vi "Lift Cycles.vi"(8 "liftMot":bool, 10 "changeDesired":bool) -> ()   [LabVIEW 2014]
uses:
  Robot Global Data.vi
  <vilib>/Rock Robotics/Network Tables/SD Write Number.vi
panel:
  in  "Desired Encoder In":dbl
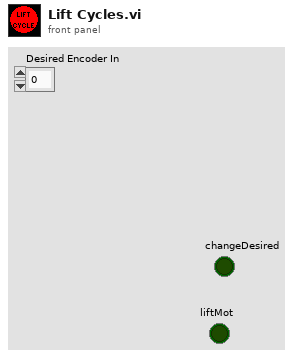
[diagram p1: front panel]
types:
  T1 = typedef "WPI_EncoderDevRef.ctl" = cluster{"DevStatus":errorcluster, "EncoderIndex":T2, "CounterIndex":T3, "DistancePerCount":dbl, "Decoding Type":T4}
  T2 = typedef "FPGA_EncoderIdx.ctl" = enum8{"Enc 0", "Enc 1", "Enc 2", "Enc 3", "Enc 4", "Enc 5", "Enc 6", "Enc 7", "Invalid"}
  T3 = typedef "FPGA_CounterCtrSystemIndex.ctl" = enum8{"Ctr 0", "Ctr 1", "Ctr 2", "Ctr 3", "Ctr 4", "Ctr 5", "Ctr 6", "Ctr 7", "Invalid"}
  T4 = typedef "WPI_EncoderType.ctl" = enum16{"1x", "2x", "4x"}
  T5 = typedef "WPI_MotorControlDeviceRef.ctl" = cluster{"DeviceStatus":errorcluster, "Type":T6, "PWM":cluster{"Controller":T7, "PWM Channel":T8, "DeadBand":T9}, "CAN":cluster{"Device Number":u8, "Control Mode":T10, "Semaphore":T11, "Max Vout":dbl, "TalonSRX Control Mode":T12}, "Invert":bool, "TransformRef":T13, "InvTransformRef":T13}
  T6 = typedef "WPI_MotorControlType.ctl" = enum16{"PWM", "CAN", "CANTalonSRX"}
  T7 = typedef "FPGA_TypedefDigitalModule.ctl" = enum16{"Controller 1"}
  T8 = typedef "FPGA_DIOPWMChannel.ctl" = enum8{"PWM 0", "PWM 1", "PWM 2", "PWM 3", "PWM 4", "PWM 5", "PWM 6", "PWM 7", "PWM 8", "PWM 9", "PWM MXP 0", "PWM MXP 1", "PWM MXP 2", "PWM MXP 3", "PWM MXP 4", "PWM MXP 5", "PWM MXP 6", "PWM MXP 7", "PWM MXP 8", "PWM MXP 9", "Invalid"}
  T9 = typedef "WPI_PWMDeadband.ctl" = cluster{"Name":string, "maxPositivePwm":i32, "minPositivePwm":i32, "centerPwm":i32, "maxNegativePwm":i32, "minNegativePwm":i32, "angularRange":u16}
  T10 = typedef "WPI_CANJaguar_ControlMode.ctl" = enum8{"Percent VBus", "Current", "Speed", "Position", "Voltage"}
  T11 = typedef "Semaphore RefNum" = refnum<k1>
  T12 = typedef "WPI_CANTalonSRX_APIControlMode.ctl" = enum8{"Percent VBus", "Speed", "Position", "Slave", "Unchanged / Invalid"}
  T13 = typedef "WPI_PWMTransform_ConPane.ctl" = refnum<vi>
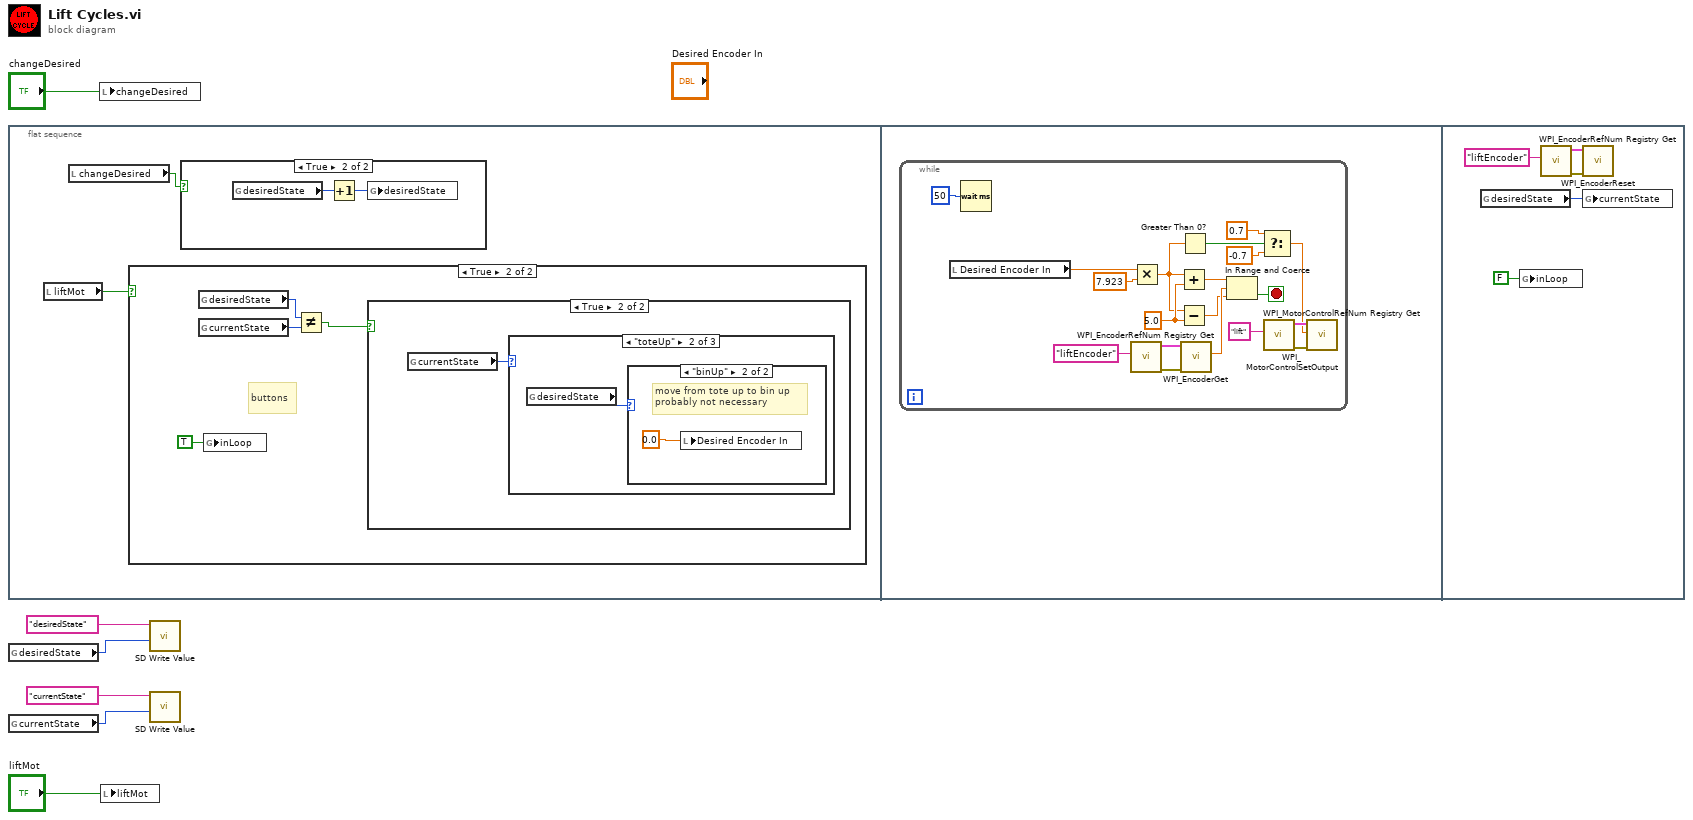
[diagram p0: block diagram]
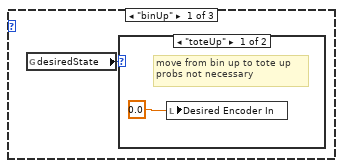
[diagram p4: hidden frame]
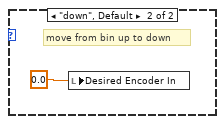
[diagram p5: hidden frame]
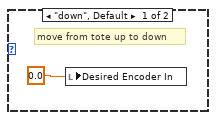
[diagram p6: hidden frame]
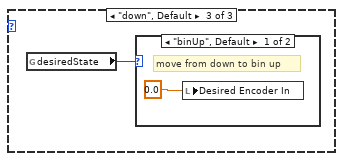
[diagram p7: hidden frame]
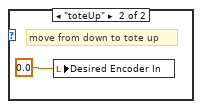
[diagram p8: hidden frame]
diagram:
  n1 = flat-sequence {
    frame #0 {
      n2 = local read "liftMot"() -> (w7:bool)
      n3 = local read "changeDesired"() -> (w8:bool)
      n4 = case shown="True" w7 {
        frame False {
        }
        frame True {
          # "buttons"
          n5 = global read "Robot Global Data.vi" "desiredState"() -> (w11:enum16{"binUp", "toteUp", "down"})
          n6 = global read "Robot Global Data.vi" "currentState"() -> (w12:enum16{"binUp", "toteUp", "down"})
          n7 = global write "Robot Global Data.vi" "inLoop"(TRUE) -> ()
          n8 = Not Equal?(x=w11, y=w12) -> (x != y?=w9:bool)
          n9 = case shown="True" w9 {
            frame False {
            }
            frame True {
              n10 = global read "Robot Global Data.vi" "currentState"() -> (w13:enum16{"binUp", "toteUp", "down"})
              n11 = case shown="\"toteUp\"" w13 {
                frame "binUp" {
                  n12 = global read "Robot Global Data.vi" "desiredState"() -> (w14:enum16{"binUp", "toteUp", "down"})
                  n13 = case shown="\"toteUp\"" w14 {
                    frame "toteUp" {
                      # "move from bin up to tote up\nprobs not necessary"
                      n14 = local write "Desired Encoder In"(0.0 ("Desired Encoder Clicks 2")) -> ()
                    }
                    frame "down", Default {
                      # "move from bin up to down"
                      n15 = local write "Desired Encoder In"(0.0 ("Desired Encoder Clicks 2")) -> ()
                    }
                  }
                }
                frame "toteUp" {
                  n16 = global read "Robot Global Data.vi" "desiredState"() -> (w17:enum16{"binUp", "toteUp", "down"})
                  n17 = case shown="\"binUp\"" w17 {
                    frame "down", Default {
                      # "move from tote up to down"
                      n18 = local write "Desired Encoder In"(0.0 ("Desired Encoder Clicks 2")) -> ()
                    }
                    frame "binUp" {
                      # "move from tote up to bin up\nprobably not necessary"
                      n19 = local write "Desired Encoder In"(0.0 ("Desired Encoder Clicks 2")) -> ()
                    }
                  }
                }
                frame "down", Default {
                  n20 = global read "Robot Global Data.vi" "desiredState"() -> (w20:enum16{"binUp", "toteUp", "down"})
                  n21 = case shown="\"binUp\", Default" w20 {
                    frame "binUp", Default {
                      # "move from down to bin up"
                      n22 = local write "Desired Encoder In"(0.0 ("Desired Encoder Clicks 2")) -> ()
                    }
                    frame "toteUp" {
                      # "move from down to tote up"
                      n23 = local write "Desired Encoder In"(0.0 ("Desired Encoder Clicks 2")) -> ()
                    }
                  }
                }
              }
            }
          }
        }
      }
      n24 = case shown="True" w8 {
        frame False {
        }
        frame True {
          n25 = global read "Robot Global Data.vi" "desiredState"() -> (w23:enum16{"binUp", "toteUp", "down"})
          n26 = Increment(x=w23) -> (x+1=w24:enum16{"binUp", "toteUp", "down"})
          n27 = global write "Robot Global Data.vi" "desiredState"(w24) -> ()
        }
      }
    }
    frame #1 {
      n28 = while {
        stop <- w36 stop-if-true
        w38 = 5.0 ("y")
        n29 = local read "Desired Encoder In"() -> (w25:dbl)
        n30 = Wait (ms)(milliseconds to wait=u32 50) -> ()  [unwired: 1 out]
        n31 = call <vilib>:"WPI_EncoderRefNum Registry Get.vi"("refnum name"="liftEncoder") -> ("error out"=w43:errorcluster, "EncoderDevRef"=w42:T1)  [unwired: 9 in]
        n32 = Multiply(x=w25, y=7.923) -> (x*y=w26:dbl)
        n33 = Add(x=w26, y=w38) -> (x+y=w39:dbl)
        n34 = Subtract(x=w26, y=w38) -> (x-y=w37:dbl)
        n35 = Greater Than 0?(x=w26) -> (x > 0?=w34:bool)
        n36 = call <vilib>:"WPI_EncoderGet.vi"("error in (no error)"=w43, "EncoderDevRef"=w42) -> ("Distance"=w40:dbl)  [unwired: 4 in, 5 out]
        n37 = In Range and Coerce(upper limit=w39, x=w40, lower limit=w37) -> (In Range?=w36:bool)  [unwired: 1 out]
        n38 = Select(t=0.7, s=w34, f=-0.7) -> (s? t:f=w28:dbl)
        n39 = call <vilib>:"WPI_MotorControlRefNum Registry Get.vi"("refnum name"="lift") -> ("error out"=w31:errorcluster, "MotorControlDevRef"=w30:T5)  [unwired: 9 in]
        n40 = call <vilib>:"WPI_MotorControlSetOutput.vi"("error in (no error)"=w31, "Output"=w28, "MotorControlDevRef"=w30) -> ()  [unwired: 6 in, 3 out]
      }
    }
    frame #2 {
      n41 = global read "Robot Global Data.vi" "desiredState"() -> (w48:enum16{"binUp", "toteUp", "down"})
      n42 = global write "Robot Global Data.vi" "inLoop"(FALSE) -> ()
      n43 = call <vilib>:"WPI_EncoderRefNum Registry Get.vi"("refnum name"="liftEncoder") -> ("error out"=w46:errorcluster, "EncoderDevRef"=w45:T1)  [unwired: 9 in]
      n44 = call <vilib>:"WPI_EncoderReset.vi"("error in (no error)"=w46, "EncoderDevRef"=w45) -> ()  [unwired: 8 in, 2 out]
      n45 = global write "Robot Global Data.vi" "currentState"(w48) -> ()
    }
  }
  n46 = global read "Robot Global Data.vi" "desiredState"() -> (w4:enum16{"binUp", "toteUp", "down"})
  n47 = global read "Robot Global Data.vi" "currentState"() -> (w1:enum16{"binUp", "toteUp", "down"})
  n48 = local write "changeDesired"("changeDesired") -> ()
  n49 = local write "liftMot"("liftMot") -> ()
  n50 = call-poly <vilib>:"SD Write Value.vi"("Numeric"=w4, "Name"="desiredState") -> ()  [unwired: 8 in, 2 out]
  n51 = call-poly <vilib>:"SD Write Value.vi"("Numeric"=w1, "Name"="currentState") -> ()  [unwired: 8 in, 2 out]
